vi "AlazarInputControl.vi"(0 "Handle":u64, 1 "Channel":u8(ring)=1 items=["A"=1, "B"=2, "C"=4, "D"=8], 2 "Coupling":u32(ring)=2 items=["AC"=1, "DC"=2], 3 "Range":u32(ring)=10 items=["20 mV"=1, "40 mV"=2, "50 mV"=3, "80 mV"=4, "100 mV"=5, "200 mV"=6, "400 mV"=7, "500 mV"=8, "800 mV"=9, "1 V"=10, "1.25 V"=33, "2 V"=11, "4 V"=12, "5 V"=13, "8 V"=14, "10 V"=15, "20 V"=16], 4 "Impedance":u32(ring)=2 items=["1 MOhm"=1, "50 Ohm"=2, ""=0], 5 "error in (no error)":errorcluster) -> (14 "Handle":u64, 18 "Return Code":u32, 19 "error out":errorcluster)   [LabVIEW 2023]
doc: "Select the input coupling, range, and impedance of a digitizer channel."
uses:
  ATSApi.dll
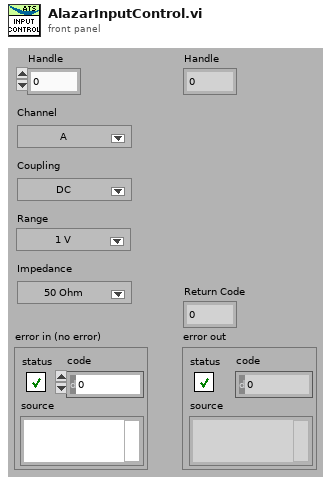
[diagram p1: front panel]
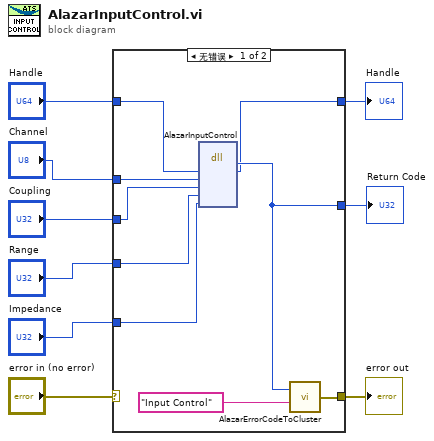
[diagram p0: block diagram]
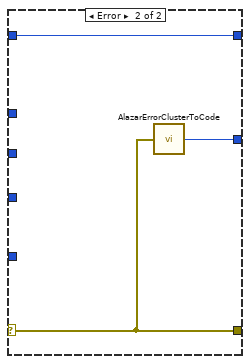
[diagram p2: hidden frame]
diagram:
  n1 = case shown="无错误" "error in (no error)" {
    selector: "error in (no error)" -> [_ w21]
    tunnel: [w15 w21] -> w8
    tunnel: [w17 w20] -> w7
    tunnel: "Handle" -> [w18 w19]
    tunnel: [w14 w19] -> w5
    tunnel: "Coupling" -> [w11 _]
    tunnel: "Range" -> [w12 _]
    tunnel: "Impedance" -> [w13 _]
    tunnel: "Channel" -> [w10 _]
    frame No Error {
      n2 = dll-call lib="ATSApi.dll" fn="AlazarInputControl"("handle"=w18, "channelID"=w10, "couplingID"=w11, "rangeID"=w12, "ImpedanceID"=w13) -> ("return type"=w17:u32, "handle"=w14:u64)  [unwired: 7 in, 2 out]
      n3 = call "AlazarErrorCodeToCluster.vi"("Message"="Input Control", "Error Code"=w17) -> ("error out"=w15:errorcluster)
    }
    frame Error {
      n4 = call "AlazarErrorClusterToCode.vi"("error in (no error)"=w21) -> ("Error Code"=w20:u32)
    }
  }
  "Handle" <- w5
  "error out" <- w8
  "Return Code" <- w7
